vi "Decorate.vi"(8 "error in (no error)":errorcluster, 10 "To be decorated":refnum<class "Testable.lvclass">, 11 "Base Decorator in":refnum<class "Base Decorator.lvclass">) -> (0 "error out":errorcluster, 3 "Base Decorator out":refnum<class "Base Decorator.lvclass">)   [LabVIEW 2020, in "Base Decorator.lvclass"]
uses:
  Base Decorator.lvclass
  Testable/Testable.lvclass
  Base Decorator.lvclass/Base Decorator.ctl
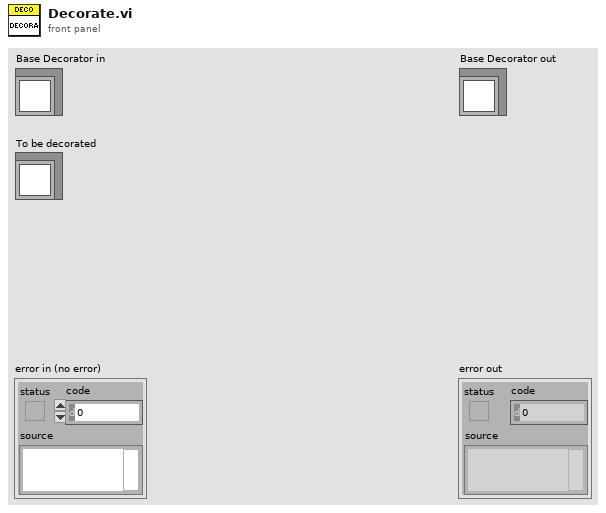
[diagram p1: front panel]
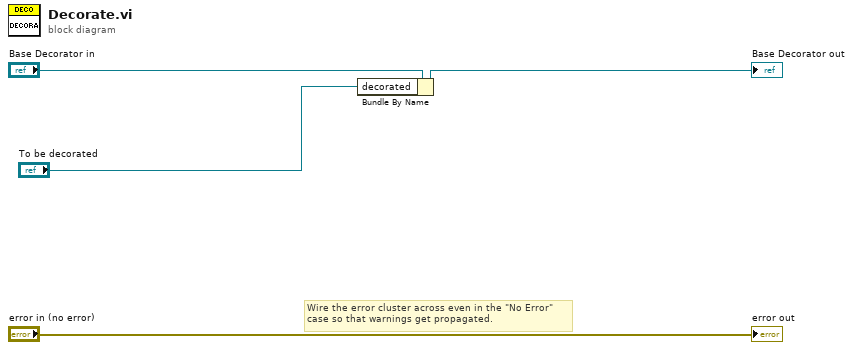
[diagram p0: block diagram]
diagram:
  # "Wire the error cluster across even in the \"No Error\"\ncase so that warnings get propagated."
  n1 = Bundle By Name(cluster="Base Decorator in", "decorated"="To be decorated") -> (→"Base Decorator out":refnum<class "Base Decorator.lvclass">)
  "error out" <- "error in (no error)"
